vi "Draw Selection.vi"(8 "Error In":errorcluster, 10 "Tree Path":string[](array[string]), 11 "WAD Cluster IN":T1) -> (0 "Error Out":errorcluster, 2 "2D Picture":picture, 3 "WAD Cluster OUT":T1)   [LabVIEW 2017]
uses:
  WAD_MainCluster.ctl
  TextureList.ctl
  PatchList.ctl
  Lumps.ctl
  <vilib>/picture/picture.llb/Draw 8-Bit Pixmap.vi
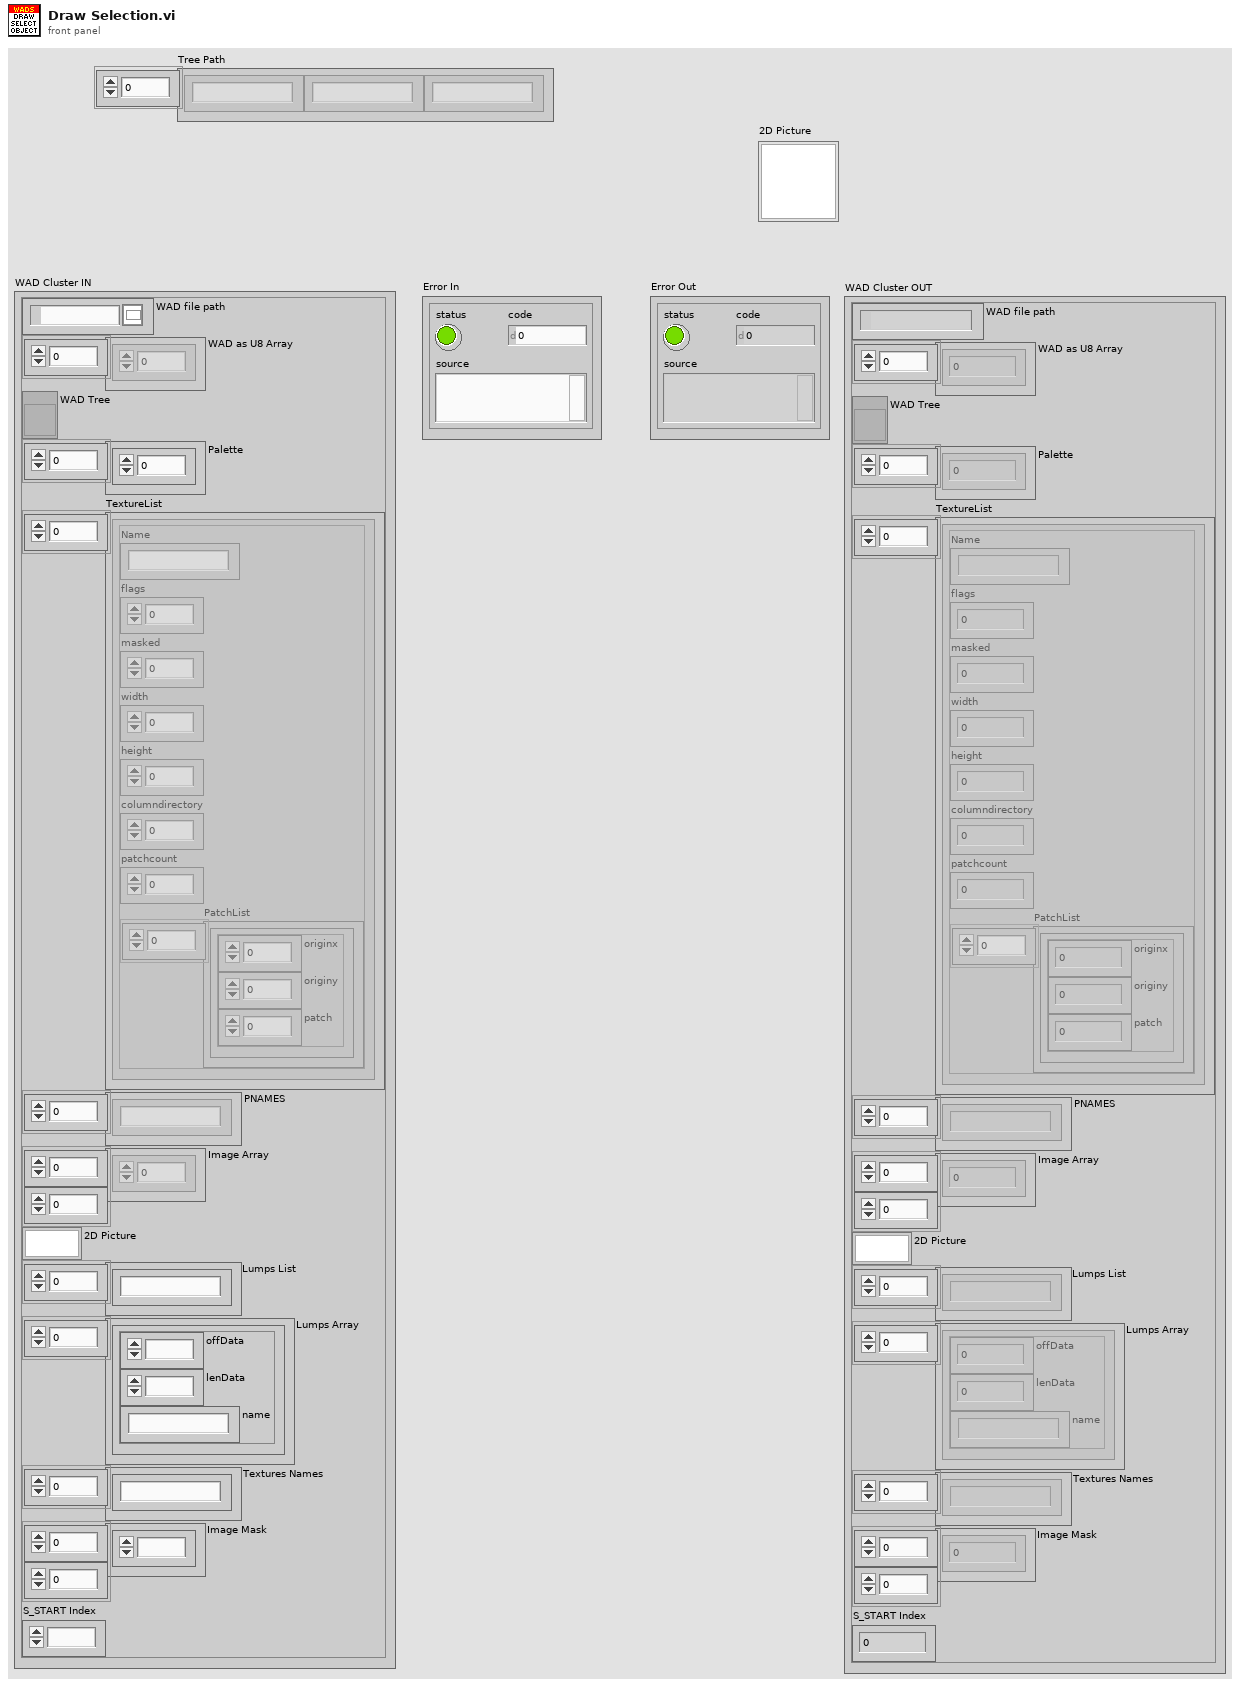
[diagram p1: front panel]
types:
  T1 = typedef "WAD_MainCluster.ctl" = cluster{"WAD file path":path, "WAD as U8 Array":u8[], "WAD Tree":refnum<vi>, "Palette":u32[], "TextureList":T2[], "PNAMES":string[], "Image Array":i16[][], "2D Picture":picture, "Lumps List":string[], "Lumps Array":T4[], "Textures Names":string[], "Image Mask":i16[][], "S_START Index":i32}
  T2 = typedef "TextureList.ctl" = cluster{"Name":string, "flags":u16, "masked":i16, "width":i16, "height":i16, "columndirectory":u32, "patchcount":i16, "PatchList":T3[]}
  T3 = typedef "PatchList.ctl" = cluster{"originx":i16, "originy":i16, "patch":i16}
  T4 = typedef "Lumps.ctl" = cluster{"offData":i32, "lenData":i32, "name":string}
  T5 = cluster{"Font Name:":string, "Size":i16, "Strikeout?":bool, "Italic?":bool, "Underline?":bool, "Outline?":bool, "Shadow?":bool, "Bold?":bool}
  T6 = typedef "PatchHeader.ctl" = cluster{"Width":u16, "Height":u16, "XOffset":i16, "YOffset":i16}
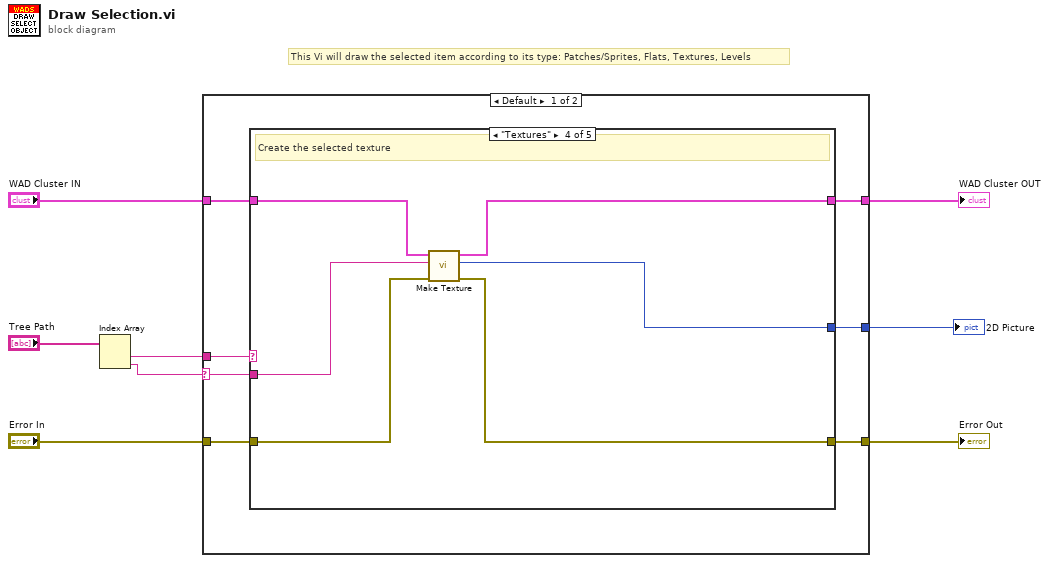
[diagram p0: block diagram]
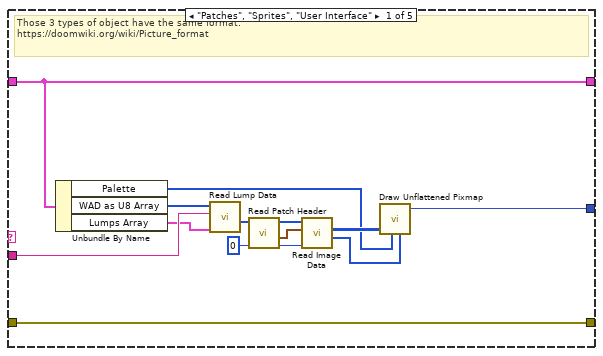
[diagram p2: hidden frame]
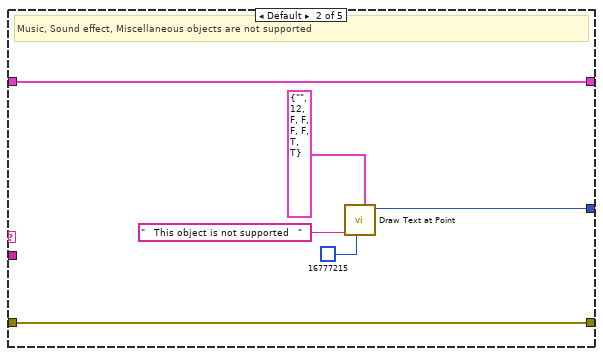
[diagram p3: hidden frame]
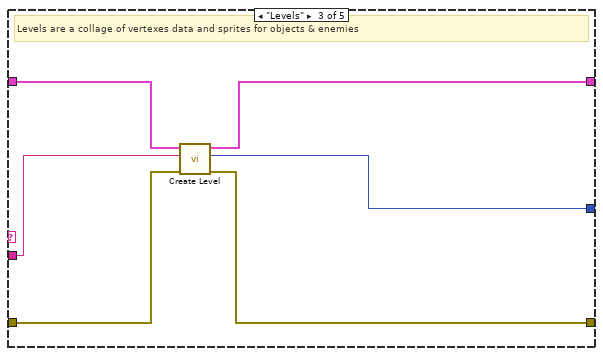
[diagram p4: hidden frame]
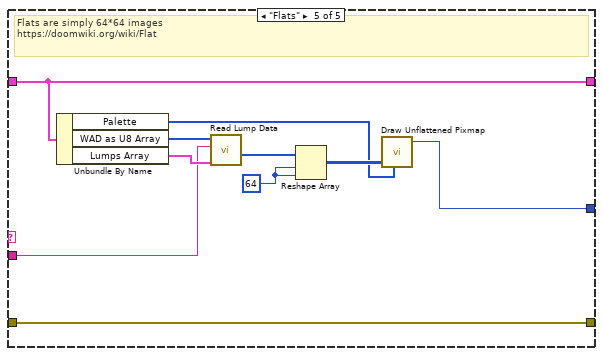
[diagram p5: hidden frame]
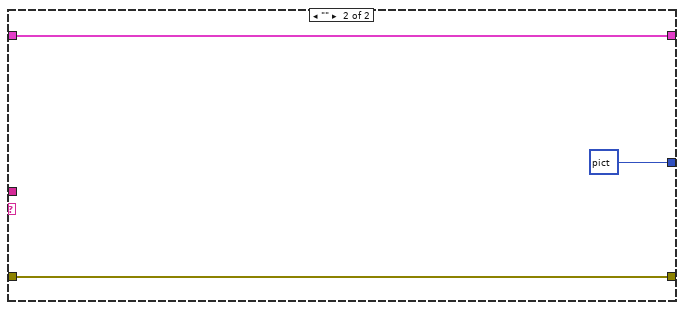
[diagram p6: hidden frame]
diagram:
  # "This Vi will draw the selected item according to its type: Patches/Sprites, Flats, Textures, Levels"
  n1 = Index Array(array="Tree Path") -> (element #1=w7:string, element #2=w2:string)  [unwired: 2 in]
  n2 = case shown="Default" w2 {
    selector: w2 -> [w10 _]
    tunnel: w7 -> [w15 _]
    tunnel: "WAD Cluster IN" -> [w14 w60]
    tunnel: [w13 w60] -> w5
    tunnel: "Error In" -> [w12 w59]
    tunnel: [w11 w59] -> w3
    tunnel: [w9 picture data[5B] ("new picture")] -> w1
    frame Default {
      n3 = case shown="\"Textures\"" w15 {
        tunnel: w14 -> [w21 w35 w41 w47 w52]
        tunnel: [w21 w35 w40 w44 w52] -> w13
        tunnel: w12 -> [w17 w32 w39 w45 w48]
        tunnel: [w17 w32 w37 w43 w48] -> w11
        tunnel: w10 -> [w28 _ w38 w46 w55]
        tunnel: [w16 w33 w36 w42 w49] -> w9
        frame "Patches", "Sprites", "User Interface" {
          # "Those 3 types of object have the same format:\nhttps://doomwiki.org/wiki/Picture_format"
          n4 = Unbundle By Name(w21) -> ("Palette"=w18:u32[], "WAD as U8 Array"=w29:u8[], "Lumps Array"=w27:T4[])
          n5 = call "Read Lump Data.vi"("Lumps Directory IN"=w27, "Lump Name"=w28, "Input U8"=w29) -> ("Lump DATA OUT"=w26:u8[])  [unwired: 5 in, 3 out]
          n6 = call "Read Patch Header.vi"("Index"=u32 0, "Patch DATA IN"=w26) -> ("Index+8"=w24:u32, "PatchHeader"=w23:T6, "Patch DATA OUT"=w25:u8[])  [unwired: 7 in]
          n7 = call "Read Image Data.vi"("Input Index"=w24, "PatchHeader"=w23, "Patch DATA IN"=w25) -> ("Mask OUT"=w19:u8[], "Image OUT"=w20:u8[][])  [unwired: 5 in, 2 out]
          n8 = call-poly <vilib>:"Draw Unflattened Pixmap.vi"("data"=w20, "color table"=w18, "mask"=w19) -> ("new picture"=w16:picture)  [unwired: 6 in]
        }
        frame Default {
          # "Music, Sound effect, Miscellaneous objects are not supported"
          n9 = call <vilib>:"Draw Text at Point.vi"("[user-specified font]"=T5 {"Font Name:"="", "Size"=12, "Strikeout?"=FALSE, "Italic?"=FALSE, "Underline?"=FALSE, "Outline?"=FALSE, "Shadow?"=TRUE, "Bold?"=TRUE}, "text color(black)"=u32 16777215, "text"="   This object is not supported   " ("String")) -> ("new picture"=w33:picture)  [unwired: 7 in, 1 out]
        }
        frame "Levels" {
          # "Levels are a collage of vertexes data and sprites for objects & enemies"
          n10 = call "Create Level.vi"("Error In"=w39, "Selected Level"=w38, "WAD Cluster IN"=w41) -> ("Error Out"=w37:errorcluster, "2D Picture"=w36:picture, "WAD Cluster OUT"=w40:T1)  [unwired: 6 in]
        }
        frame "Textures" {
          # "Create the selected texture"
          n11 = call "Make Texture.vi"("Error In"=w45, "Texture Name"=w46, "WAD Cluster IN"=w47) -> ("Error Out"=w43:errorcluster, "2D Picture"=w42:picture, "WAD Cluster OUT"=w44:T1)  [unwired: 6 in]
        }
        frame "Flats" {
          w53 = 64
          # "Flats are simply 64*64 images\nhttps://doomwiki.org/wiki/Flat"
          n12 = Unbundle By Name(w52) -> ("Palette"=w50:u32[], "WAD as U8 Array"=w57:u8[], "Lumps Array"=w56:T4[])
          n13 = call "Read Lump Data.vi"("Lumps Directory IN"=w56, "Lump Name"=w55, "Input U8"=w57) -> ("Lump DATA OUT"=w54:u8[])  [unwired: 5 in, 3 out]
          n14 = Reshape Array(w54, w53, w53) -> (w51:u8[][])
          n15 = call-poly <vilib>:"Draw Unflattened Pixmap.vi"("data"=w51, "color table"=w50) -> ("new picture"=w49:picture)  [unwired: 7 in]
        }
      }
    }
    frame "" {
    }
  }
  "WAD Cluster OUT" <- w5
  "Error Out" <- w3
  "2D Picture" <- w1
